vi "PH_AWG-510.destructor.vi"(0 "i ref in":refnum<vi>, 5 "error in":errorcluster) -> (19 "error out":errorcluster)   [LabVIEW 2014, in "PH_AWG-510.lvlib"]
doc: "This is the destructor of a class.\n\nLicense Agreement for this software:\n\nCopyright (C)\nGesellschaft für Schwerionenforschung, GSI\nPlanckstr. 1\n64291 Darmstadt\nGermany\n\nContact: D.Beck@gsi.de \n\nThis program is free software; you can redistribute it and/or modify it under the terms of the \nGNU General Public License as published by the Free Software Foundation; either version 2 of \nthe license, or (at your option) any later version.\n\nThis program is distributed in the hope that it will be useful, but WITHOUT ANY WARRANTY; \nwithout even the implied warranty of MERCHANTABILITY or FITNESS FOR A PARTICULAR PURPOSE. See the GNU General License for more details (http://www.gnu.org).\n\nGesellschaft für Schwerionenforschung, GSI\nPlanckstr. 1, 64291 Darmstadt, Germany\nFor all questions and ideas contact: M.Richter@gsi.de, H.Brand@gsi.de or D.Beck@gsi.de.\nLast update: 16-JUN-2004"
uses:
  PH_AWG-510.lvlib
  PH_PSDBWriter/PH_PSDBWriter.lvlib
  PH_StatusHandler/PH_StatusHandler.lvlib
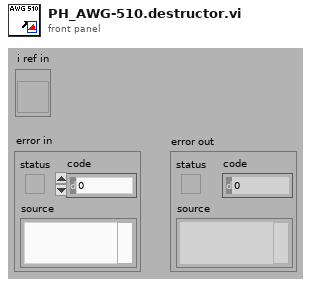
[diagram p1: front panel]
types:
  T1 = enum16{"SetAttribute", "GetAttribute", "CreateAttribute", "DestroyAttribute", "DestroyAllAtributes"}
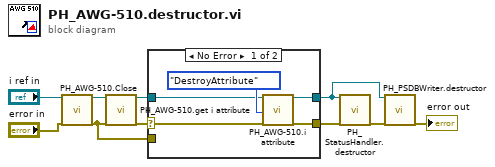
[diagram p0: block diagram]
diagram:
  n1 = call "PH_AWG-510.Close.vi"("VI in"="i ref in", "error in (no error)"="error in") -> ("VI out"=w6:refnum<vi>, "error out"=w1:errorcluster)  [unwired: 16 in]
  n2 = call "PH_AWG-510.get i attribute.vi"("i ref in"=w6, "error in (no error)"=w1) -> ("i ref out"=w9:refnum<vi>, "error out"=w2:errorcluster)  [unwired: 15 in, 1 out]
  n3 = case shown="No Error" w2 {
    selector: w2 -> [w11 _]
    tunnel: [w14 w17] -> w10
    tunnel: w9 -> [w13 w16]
    tunnel: [w12 w16] -> w3
    tunnel: w1 -> [_ w17]
    frame No Error {
      n4 = call "PH_AWG-510.i attribute.vi"("VI Refnum"=w13, "Action"=T1."DestroyAttribute", "error in (no error)"=w11) -> ("VI Refnum out"=w12:refnum<vi>, "error out"=w14:errorcluster)  [unwired: 14 in, 1 out]
    }
    frame Error {
    }
  }
  n5 = call "PH_StatusHandler.destructor.vi"("i ref in"=w3, "error in(no error)"=w10) -> ("error out"=w4:errorcluster)  [unwired: 17 in]
  n6 = call "PH_PSDBWriter.destructor.vi"("i ref in"=w3, "error in(no error)"=w4) -> ("error out"=→"error out":errorcluster)  [unwired: 17 in]
